vi "RUN_hlo.vi"(8 "error in (no error)":errorcluster) -> (0 "error out":errorcluster, 3 "String out":string)   [LabVIEW 2021]
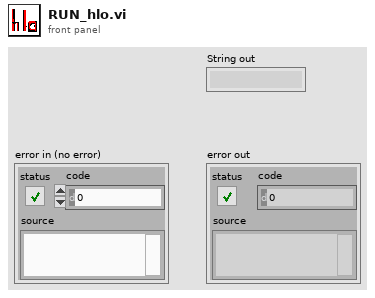
[diagram p1: front panel]
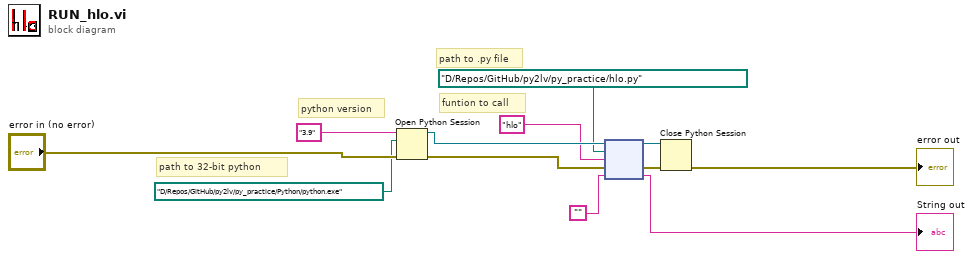
[diagram p0: block diagram]
diagram:
  # "funtion to call"
  # "path to .py file"
  # "python version"
  # "path to 32-bit python"
  n1 = Open Python Session(python version="3.9", python path=path "D:/Repos/GitHub/py2lv/py_practice/Python/python.exe", 3:"error in (no error)") -> (session out=w4:refnum<k35>, error out=w6:errorcluster)
  n2 = node(w4, path "D:/Repos/GitHub/py2lv/py_practice/hlo.py", "hlo", w6, "") -> (w5:refnum<k35>, w7:errorcluster, →"String out":string)  [unwired: 2 out]
  n3 = Close Python Session(session in=w5, error in=w7) -> (11:→"error out":errorcluster)
